vi "Get Number 2 Digit 3.vi"(10 "Digit 2":string, 11 "Array":string[][](array[string])) -> (2 "Pattern number 2":string, 3 "Digit 3":string)   [LabVIEW 2019, in "Day 8.lvlib"]
uses:
  Day 8.lvlib
panel:
  out "Array 2":string[](array[string])
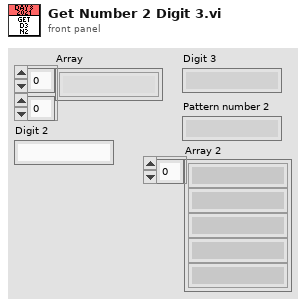
[diagram p1: front panel]
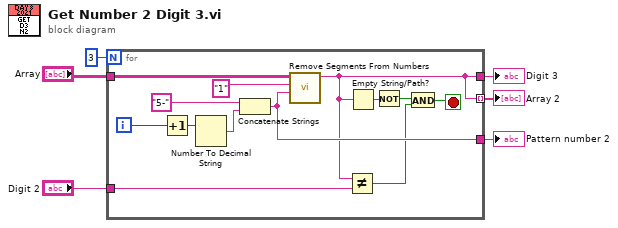
[diagram p0: block diagram]
diagram:
  n1 = for {
    N: 3 -> [_]
    tunnel: "Array" -> [w19]
    tunnel: [w10] -> w4
    tunnel: [w14] -> w5
    tunnel: "Digit 2" -> [w11]
    tunnel: [w10] -> w1 mode=indexing
    i -> [w15]
    stop <- w7 stop-if-true
    n2 = Increment(x=w15) -> (x+1=w16:i32)
    n3 = Number To Decimal String(number=w16) -> (decimal integer string=w17:string)  [unwired: 1 in]
    n4 = Concatenate Strings("5-" ("Pattern For Number Of Letters A"), w17) -> (w14:string)
    n5 = call "Remove Segments From Numbers.vi"("Pattern For Letter Of Letters B"=w14, "Pattern For Number Of Letters A"="1", "Array"=w19) -> ("Result"=w10:string)  [unwired: 8 in]
    n6 = Not Equal?(x=w10, y=w11) -> (x != y?=w8:bool)
    n7 = Empty String/Path?(string/path=w10) -> (empty?=w12:bool)
    n8 = Not(x=w12) -> (.not. x?=w9:bool)
    n9 = And(x=w9, y=w8) -> (x .and. y?=w7:bool)
  }
  "Pattern number 2" <- w5
  "Digit 3" <- w4
  "Array 2" <- w1
